vi "VoltageInputSetSensorType.vi"(0 "error in (no error)":errorcluster, 2 "Sensor Type":u32(ring) items=["SENSOR_TYPE_VOLTAGE"=0, "SENSOR_TYPE_1114"=11140, "SENSOR_TYPE_1117"=11170, "SENSOR_TYPE_1123"=11230, "SENSOR_TYPE_1127"=11270, "SENSOR_TYPE_1130_PH"=11301, "SENSOR_TYPE_1130_ORP"=11302, "SENSOR_TYPE_1132"=11320, "SENSOR_TYPE_1133"=11330, "SENSOR_TYPE_1135"=11350, "SENSOR_TYPE_1142"=11420, "SENSOR_TYPE_1143"=11430, "SENSOR_TYPE_3500"=35000, "SENSOR_TYPE_3501"=35010, "SENSOR_TYPE_3502"=35020, "SENSOR_TYPE_3503"=35030, "SENSOR_TYPE_3507"=35070, "SENSOR_TYPE_3508"=35080, "SENSOR_TYPE_3509"=35090, "SENSOR_TYPE_3510"=35100, "SENSOR_TYPE_3511"=35110, "SENSOR_TYPE_3512"=35120, "SENSOR_TYPE_3513"=35130, "SENSOR_TYPE_3514"=35140, "SENSOR_TYPE_3515"=35150, "SENSOR_TYPE_3516"=35160, "SENSOR_TYPE_3517"=35170, "SENSOR_TYPE_3518"=35180, "SENSOR_TYPE_3519"=35190, "SENSOR_TYPE_3584"=35840, "SENSOR_TYPE_3585"=35850, "SENSOR_TYPE_3586"=35860, "SENSOR_TYPE_3587"=35870, "SENSOR_TYPE_3588"=35880, "SENSOR_TYPE_3589"=35890, "SENSOR_TYPE_ADP1000_PH"=110000, "SENSOR_TYPE_ADP1000_ORP"=110001], 3 "Device In":u64) -> (7 "error out":errorcluster, 10 "Device Out":u64)   [LabVIEW 2020, in "Phidget Voltage Input.lvlib"]
doc: "${SensorType:Header}"
uses:
  <instrlib>/Phidgets/Phidget Voltage Input/Phidget Voltage Input.lvlib
  <instrlib>/Phidgets/Phidget Common/Phidget Common.lvlib
  phidget22.dll
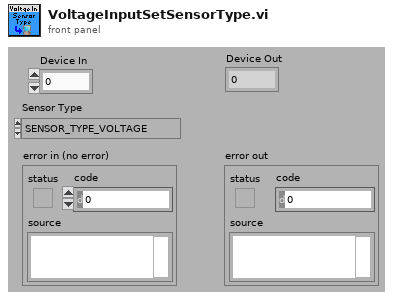
[diagram p1: front panel]
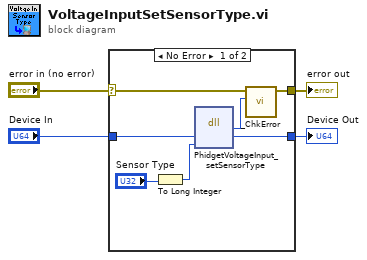
[diagram p0: block diagram]
diagram:
  n1 = case shown="No Error" "error in (no error)" {
    selector: "error in (no error)" -> [w9 w13]
    tunnel: [w8 w13] -> w3
    tunnel: "Device In" -> [w11 w12]
    tunnel: [w10 w12] -> w1
    frame No Error {
      n2 = To Long Integer(number="Sensor Type") -> (32bit integer=w5:i32)
      n3 = dll-call lib="phidget22.*" fn="PhidgetVoltageInput_setSensorType"("phid"=w11, "interval"=w5) -> ("return type"=w7:i32, "phid"=w10:u64)  [unwired: 4 in, 2 out]
      n4 = call <instrlib>:"_ChkError.vi"("Return Code"=w7, "error in (no error)"=w9) -> ("error out"=w8:errorcluster)  [unwired: 9 in]
    }
    frame Error {
    }
  }
  "error out" <- w3
  "Device Out" <- w1
